vi "Generate Test Data.vi"(11 "MC Data in":refnum<class "MC Data.lvclass">) -> (3 "MC Data out":refnum<class "MC Data.lvclass">)   [LabVIEW 2014, in "MC Data.lvclass"]
uses:
  MC Data.lvclass
  MC Data.lvclass/MC Data.ctl
  Alicat Data.lvclass
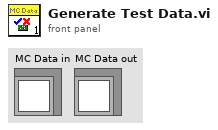
[diagram p1: front panel]
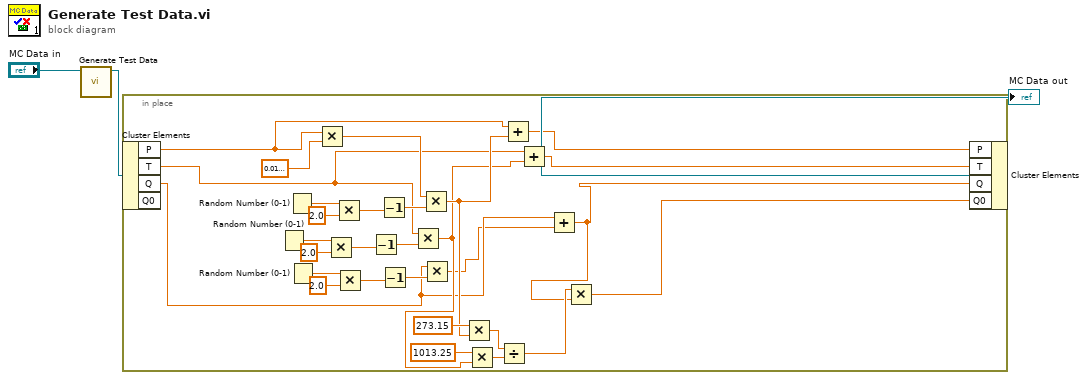
[diagram p0: block diagram]
diagram:
  n1 = call-parent "Generate Test Data.vi"("Data in"="MC Data in") -> ("Data out"=w2:refnum<class "MC Data.lvclass">)  [unwired: 10 in]
  n2 = in-place {
    n3 = in-place-cluster #1(w2) -> ("P"=w12:sgl, "T"=w9:sgl, "Q"=w6:sgl)  [unwired: 1 out]
    n4 = Random Number (0-1)() -> (number: 0 to 1=w19:dbl)
    n5 = Random Number (0-1)() -> (number: 0 to 1=w31:dbl)
    n6 = Random Number (0-1)() -> (number: 0 to 1=w23:dbl)
    n7 = Multiply(x=w12, y=sgl 0.02) -> (x*y=w27:sgl)
    n8 = Multiply(x=w19, y=2.0) -> (x*y=w21:dbl)
    n9 = Multiply(x=w31, y=2.0) -> (x*y=w29:dbl)
    n10 = Multiply(x=w23, y=2.0) -> (x*y=w25:dbl)
    n11 = Decrement(x=w21) -> (x-1=w22:dbl)
    n12 = Decrement(x=w29) -> (x-1=w28:dbl)
    n13 = Decrement(x=w25) -> (x-1=w26:dbl)
    n14 = Multiply(x=w9, y=w22) -> (x*y=w8:dbl)
    n15 = Multiply(x=w27, y=w28) -> (x*y=w11:dbl)
    n16 = Multiply(x=w6, y=w26) -> (x*y=w5:dbl)
    n17 = Multiply(x=273.15, y=w11) -> (x*y=w17:dbl)
    n18 = Multiply(x=1013.25, y=w8) -> (x*y=w15:dbl)
    n19 = Divide(x=w17, y=w15) -> (x/y=w14:dbl)
    n20 = Add(x=w12, y=w11) -> (x+y=w10:dbl)
    n21 = Add(x=w9, y=w8) -> (x+y=w7:dbl)
    n22 = Add(x=w6, y=w5) -> (x+y=w4:dbl)
    n23 = Multiply(x=w14, y=w4) -> (x*y=w13:dbl)
    n24 = in-place-cluster #1("P"=w10, "T"=w7, "Q"=w4, "Q0"=w13) -> (→"MC Data out":refnum<class "MC Data.lvclass">)
  }
